vi "ILAB_CreateFromTemplate.vi"(3 "path":string, 4 "suffix":string, 5 "templateName":string) -> (0 "viReference":refnum<vi>, 1 "name":string)   [LabVIEW 2009]
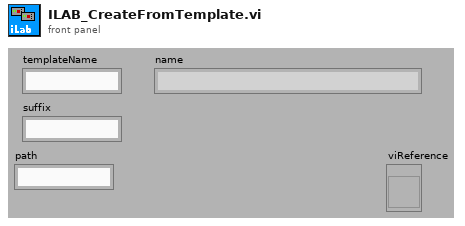
[diagram p1: front panel]
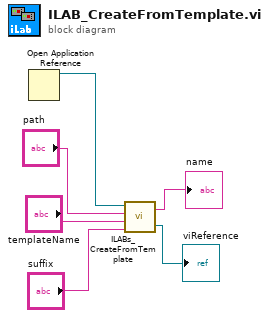
[diagram p0: block diagram]
diagram:
  n1 = Open Application Reference() -> (3:w6:refnum<vi>)  [unwired: 1 in, 4 out]
  n2 = call "ILABs_CreateFromTemplate.vi"("suffix"="suffix", "templateName"="templateName", "path"="path", "appRef"=w6) -> ("viReference"=→"viReference":refnum<vi>, "name"=→"name":string)
